vi "ToPlot.vi"(8 "error in":errorcluster, 11 "Generic in":refnum<class "Generic.lvclass">) -> (0 "error out":errorcluster, 3 "Plot out":refnum<class "Plot.lvclass">)   [LabVIEW 2014, in "Plot.lvclass"]
uses:
  Plot.lvclass
  Generic/Generic.lvclass
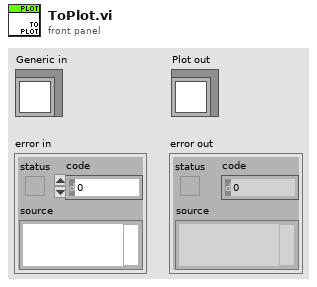
[diagram p1: front panel]
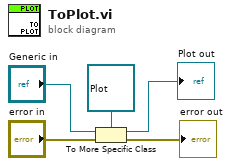
[diagram p0: block diagram]
diagram:
  n1 = To More Specific Class(target class=refnum<class "Plot.lvclass"> refnum ("RotaryColorScale in 2"), reference="Generic in", error in="error in") -> (specific class reference=→"Plot out":refnum<class "Plot.lvclass">, error out=→"error out":errorcluster)
